vi "TestFollowVI.vi"() -> ()   [LabVIEW 2016]
panel:
  out "Real":dbl
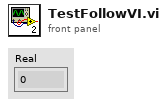
[diagram p1: front panel]
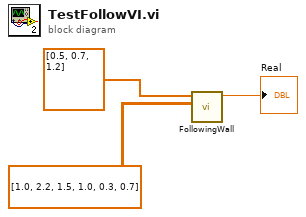
[diagram p0: block diagram]
diagram:
  n1 = call "FollowingWall.vi"("2-D Array of Real"=dbl[][] [[1.0, 2.2, 1.5], [1.0, 0.3, 0.7]], "Array - Numeric"=dbl[] [0.5, 0.7, 1.2]) -> ("theta_fw"=→"Real":dbl)  [unwired: 9 in]
